vi "Read Configuration File.vi"(8 "error in (no error)":errorcluster, 11 "Instrument in":refnum<class "Instrument.lvclass">) -> (0 "error out":errorcluster, 3 "Instrument out":refnum<class "Instrument.lvclass">)   [LabVIEW 2019, in "Instrument.lvclass"]
uses:
  Instrument.lvclass
  C:/Program Files (x86)/National Instruments/LabVIEW 2019/vi.lib/JKI/JKI SMO/SMO/SMO.lvclass
  Instrument.lvclass/Instrument.ctl
  Configuration/Configuration.lvclass/Configuration.ctl
  Configuration/Write Section.vi
  <vilib>/JKI/JKI SMO/SMO/Protected/ThisLevelClassName.vi
  Configuration/Configuration.lvclass
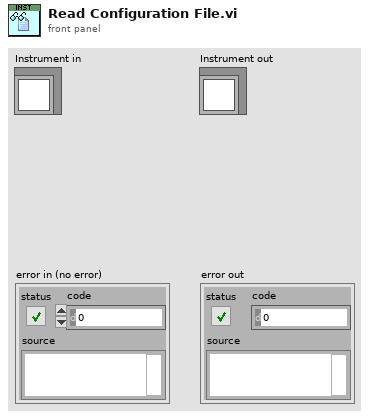
[diagram p1: front panel]
types:
  T1 = typedef "Instrument.lvclass/Configuration--Cluster.ctl" = cluster{"Hardware":T2, "SMO":T3}
  T2 = typedef "Instrument.lvclass/HW Configuration--Cluster.ctl" = cluster{"Address":string, "Type":string, "COM Type":string}
  T3 = typedef "Instrument.lvclass/SMO Configuration--Cluster.ctl" = cluster{"Address":string, "Port":u16, "RC Type":T4, "Debug Mode?":bool, "PGSQL Address":string[], "GetAll Names":string[]}
  T4 = typedef "RemoteControl.lvclass/RC Com Type--enum.ctl" = enum16{"RC", "STM", "ZMQ"}
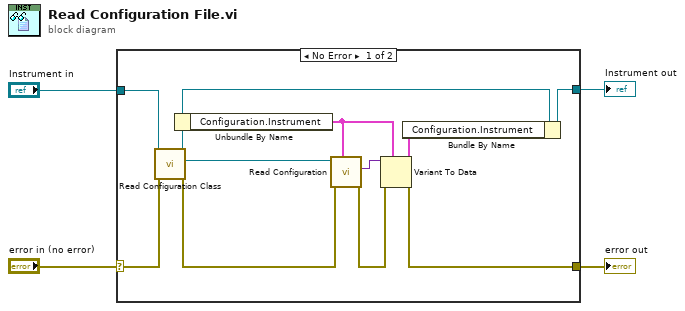
[diagram p0: block diagram]
diagram:
  n1 = case shown="No Error" "error in (no error)" {
    selector: "error in (no error)" -> [w12 w17]
    tunnel: [w11 w17] -> w4
    tunnel: [w15 w16] -> w3
    tunnel: "Instrument in" -> [w14 w16]
    frame No Error {
      n2 = call "Read Configuration Class.vi"("error in (no error)"=w12, "Instrument in"=w14) -> ("error out"=w9:errorcluster, "Configuration"=w8:refnum<class "Configuration.lvclass">, "Instrument out"=w13:refnum<class "Instrument.lvclass">)  [unwired: 7 in]
      n3 = Unbundle By Name(w13) -> ("Configuration.Instrument"=w10:T1)
      n4 = call "Read Configuration.vi"("INI Fomatted Cluster Type"=w10, "error in (no error)"=w9, "Configuration in"=w8) -> ("error out"=w6:errorcluster, "Configuration"=w7:variant)  [unwired: 6 in, 1 out]
      n5 = Variant To Data(error in=w6, type=w10, Variant=w7) -> (data=w5:T1, error out=w11:errorcluster)
      n6 = Bundle By Name(cluster=w13, "Configuration.Instrument"=w5) -> (w15:refnum<class "Instrument.lvclass">)
    }
    frame Error {
    }
  }
  "Instrument out" <- w3
  "error out" <- w4
